vi "DisplayPanel.vi"() -> ()   [LabVIEW 2013]
uses:
  MvLVLib/MvCameraControl.lvlib
panel:
  in  "TimerTriggerActivation":u16(ring) items=["RisingEdge", "FallingEdge", "AnyEdge", "LevelHigh", "LevelLow"]
  in  "TimerTriggerSoftware":bool
  in  "TimerTriggerSource":u16(ring) items=["Off", "OptoCoupledInput0", "OptoCoupledInput1", "OptoCoupledInput2", "OptoCoupledInput3", "RS422diffInput0", "RS422diffInput1", "RS422diffInput2", "RS422diffInput3", "TTLInput0", "TTLInput1", "TTLInput2", "TTLInput3", "Timer0Active", "Timer1Active", "Timer2Active", "Timer3Active", "Encoder0", "Encoder1", "SoftwareSignal0", "Continuous"]
  in  "TimerFrequency":u32
  in  "TimerDelay":u32
  in  "TimerDuration":u32
  in  "TimerSelector":u16(ring) items=["Timer0", "Timer1", "Timer2", "Timer3"]
  in  "Interface List":u16(ring)
  out "handle":u64 format="%x"
  in  "Close Interface":bool
  in  "Open Interface":bool
  in  "Enum Interface":bool
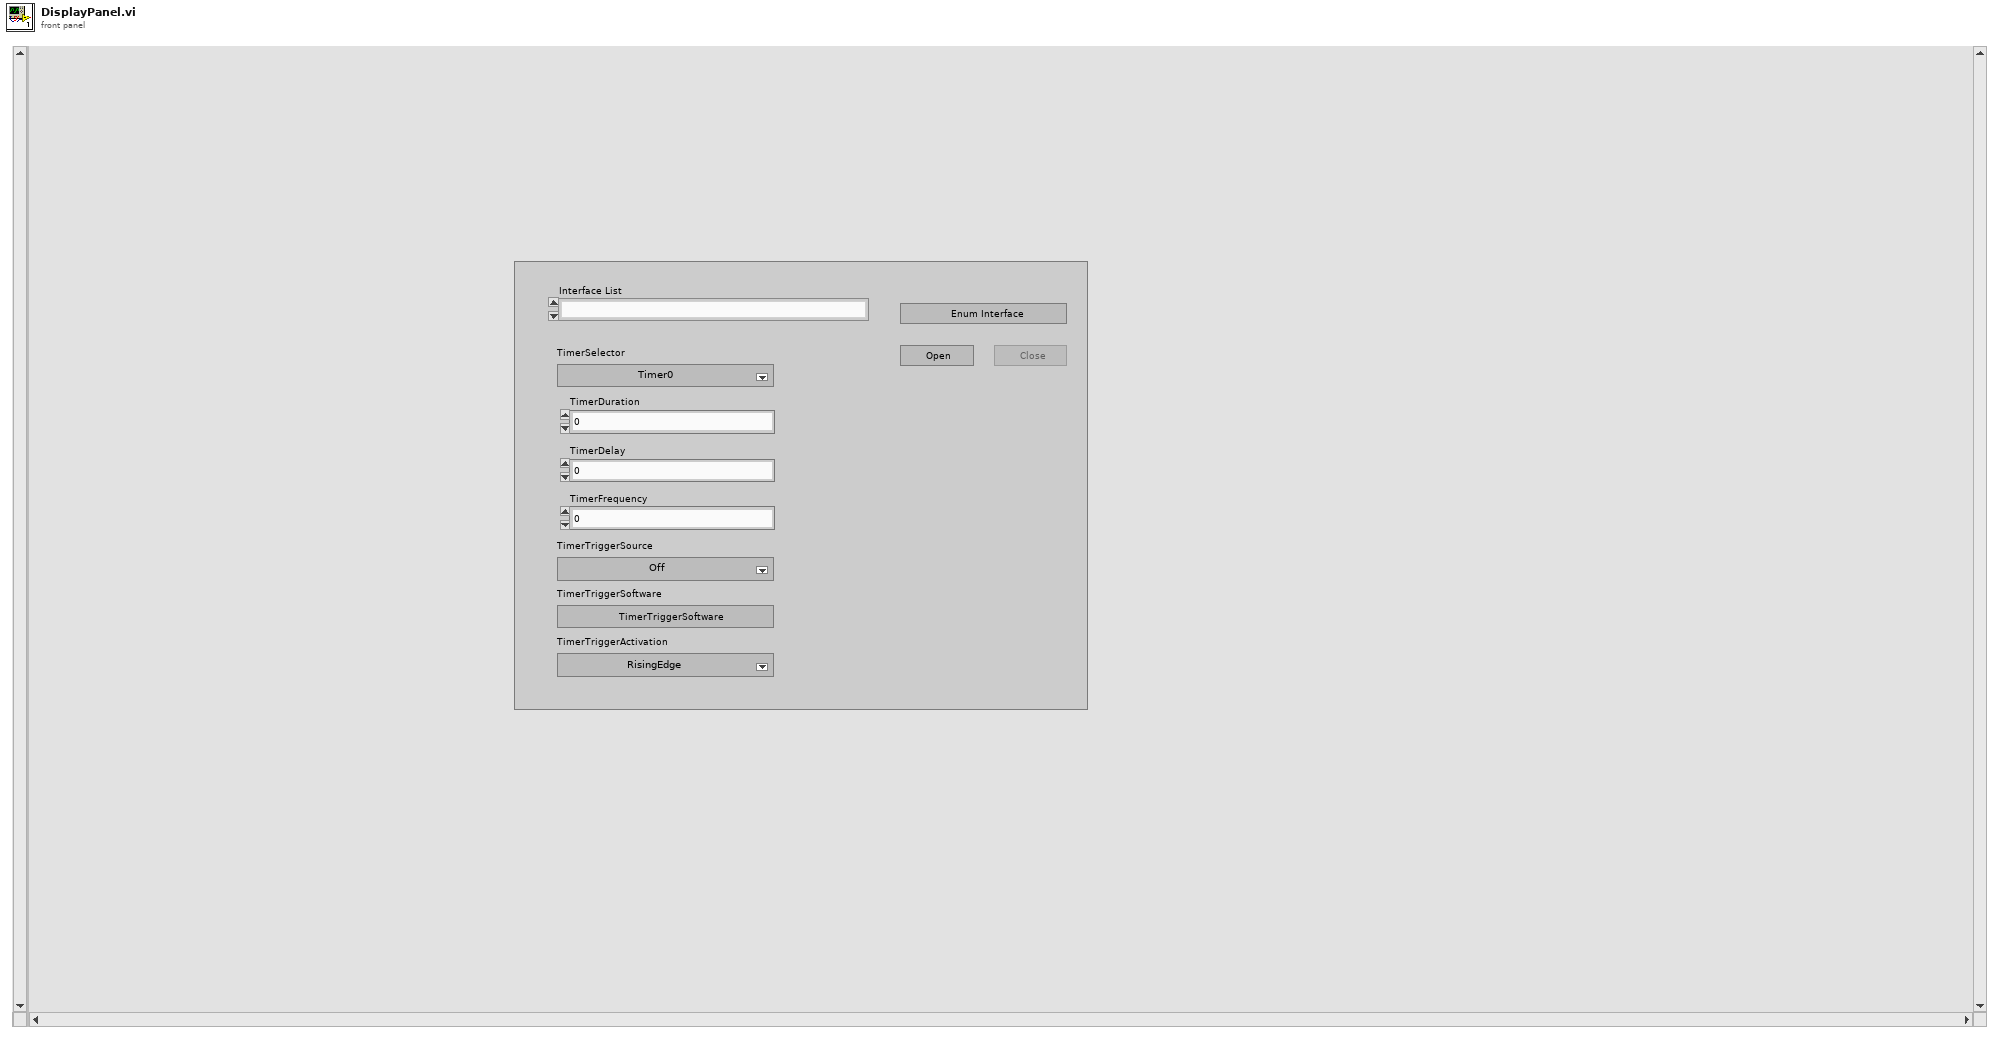
[diagram p1: front panel]
types:
  T1 = enum8{"Enabled", "Disabled", "Disabled and Grayed Out"}
  T2 = cluster{"nTLayerType":u32, "nPCIEInfo":u32, "chInterfaceID":string, "chDisplayName":string, "chSerialNumber":string, "chModelName":string, "chManufacturer":string, "chDeviceVersion":string, "chUserDefinedName":string}[]
  T3 = cluster{"nCurValue":u32, "nSupportedNum":u32, "nSupportValue":u32[], "nReserved[0]":u32, "nReserved[1]":u32, "nReserved[2]":u32, "nReserved[3]":u32}
  T4 = cluster{"nValue":u32, "chSymbolic":string, "nReserved[0]":u32, "nReserved[1]":u32, "nReserved[2]":u32, "nReserved[3]":u32}
  T5 = cluster{"nCurValue":u32, "nMax":u32, "nMin":u32, "nInc":u32, "nReserved[0]":u32, "nReserved[1]":u32, "nReserved[2]":u32, "nReserved[3]":u32}
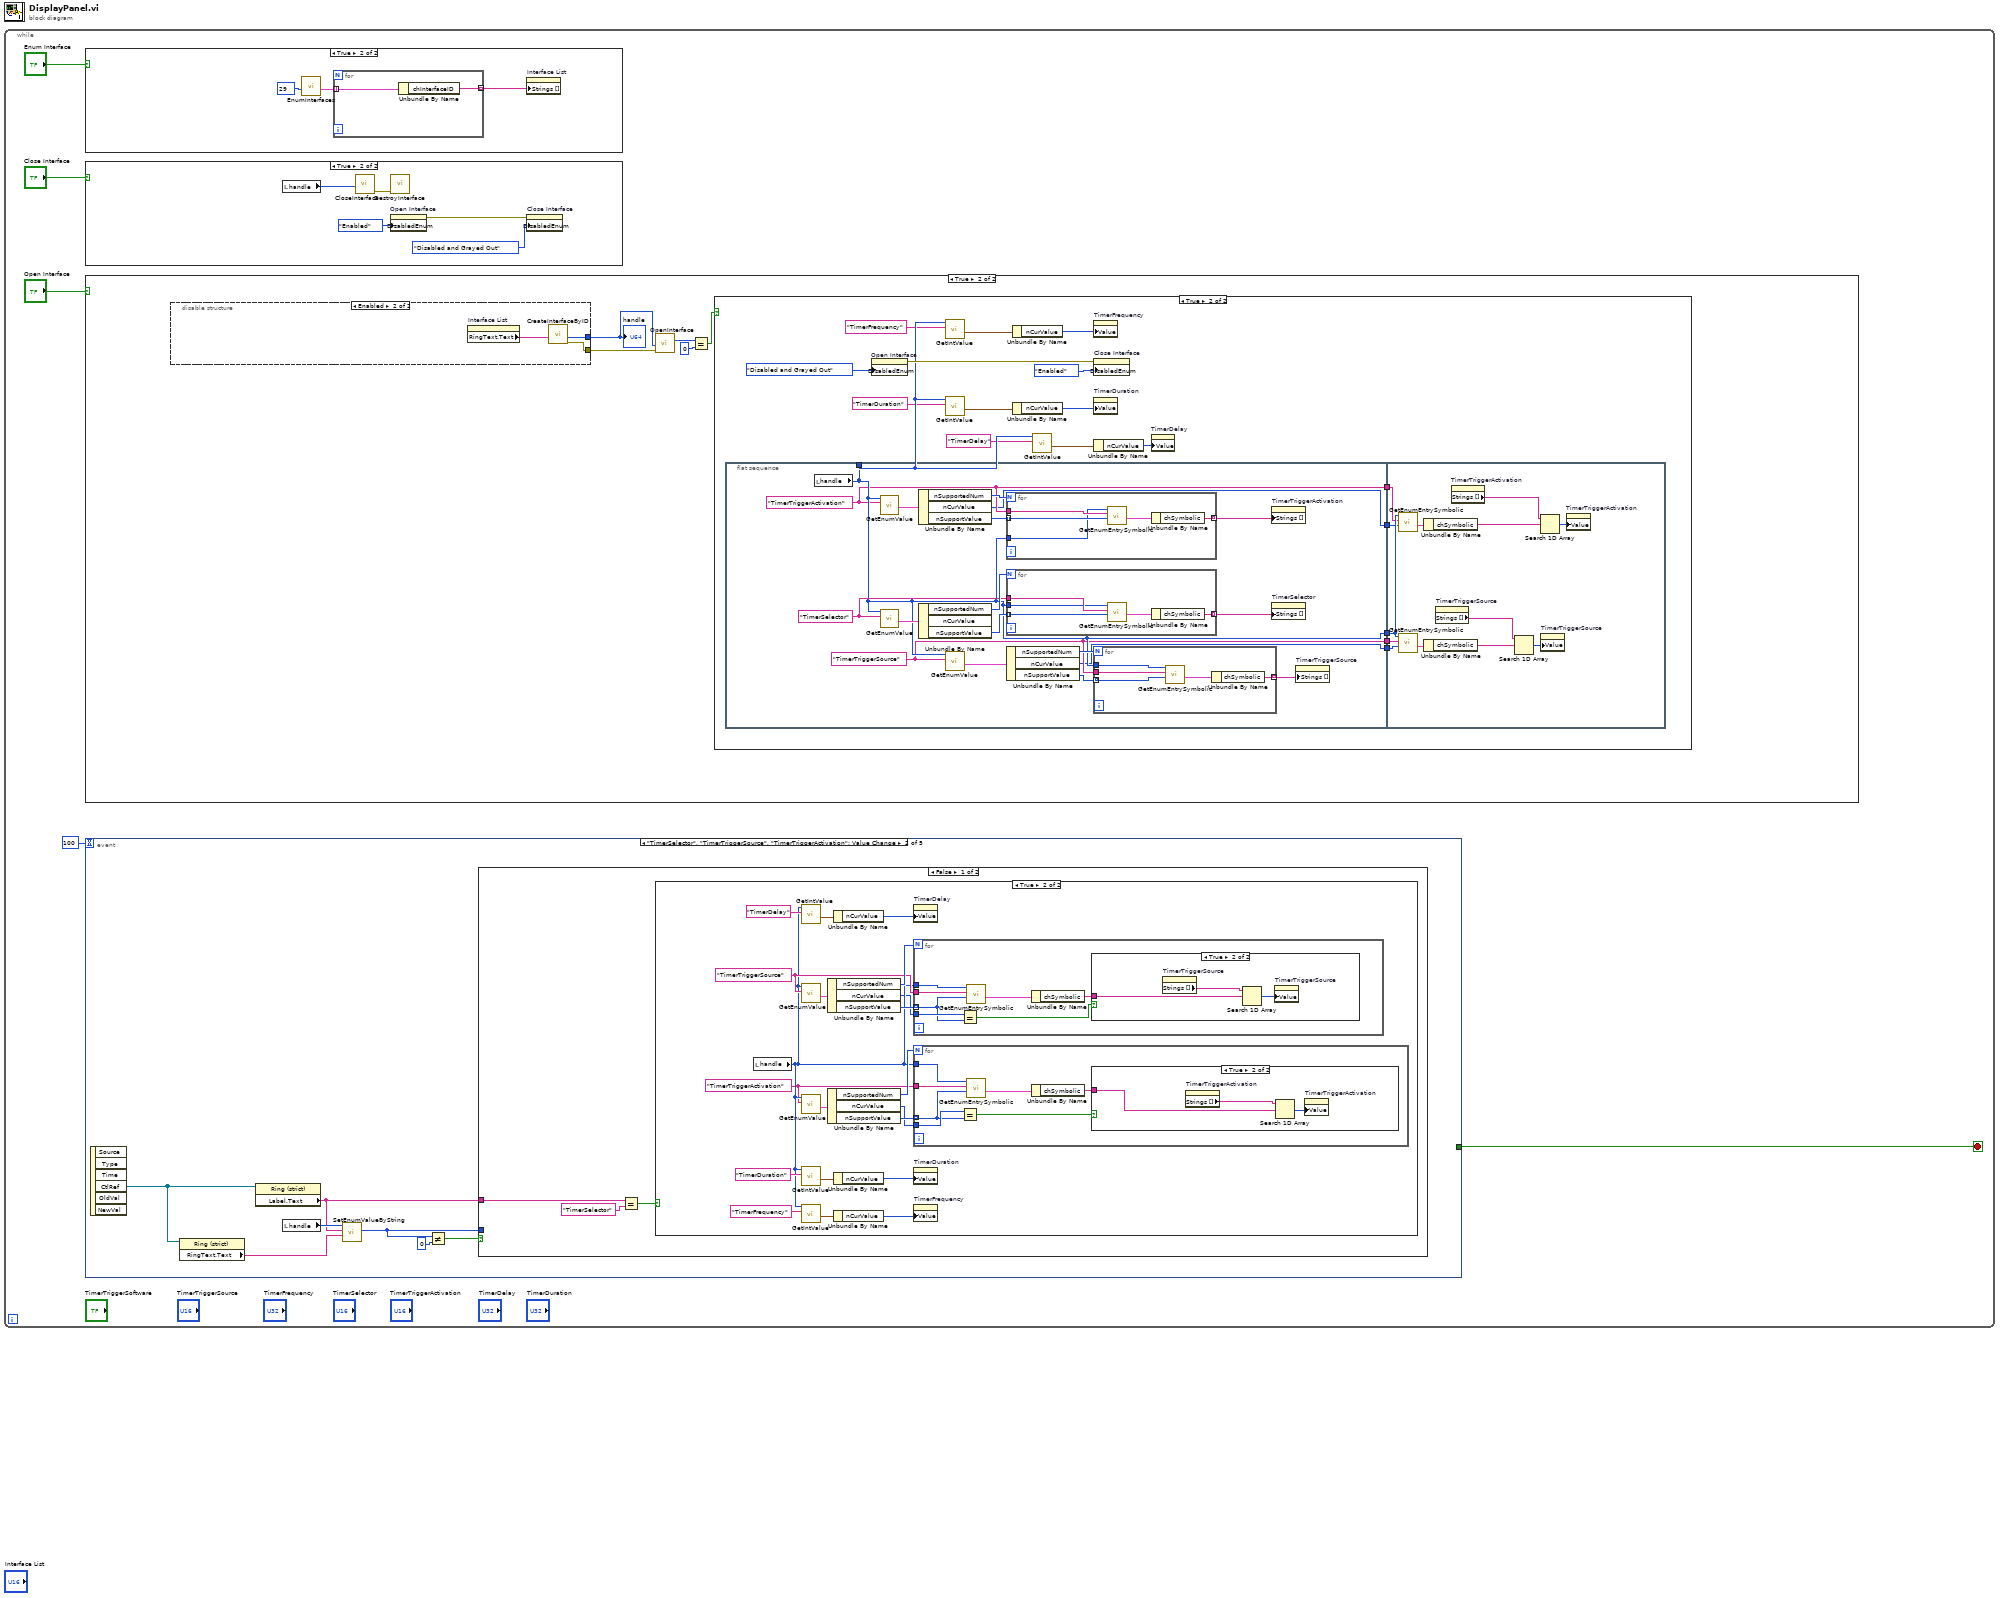
[diagram p0: block diagram]
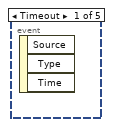
[diagram p2: hidden frame]
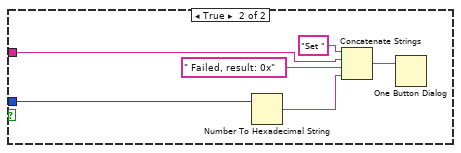
[diagram p6: hidden frame]
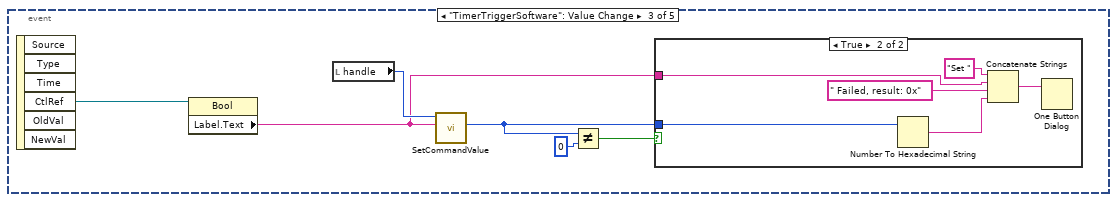
[diagram p7: hidden frame]
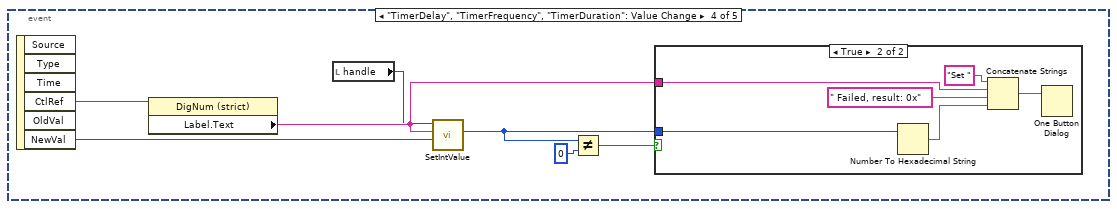
[diagram p9: hidden frame]
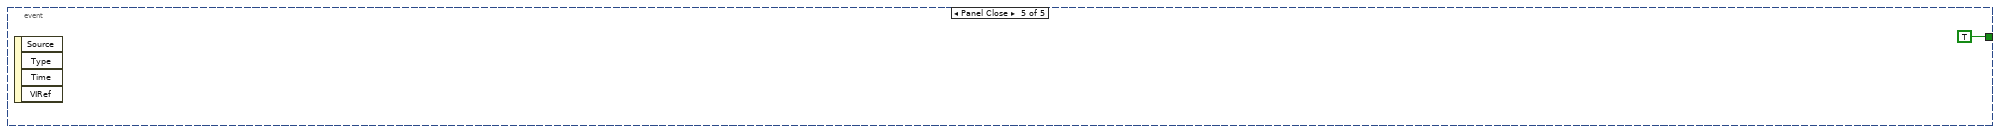
[diagram p11: hidden frame]
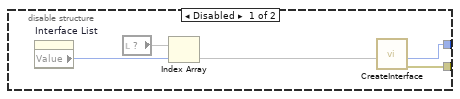
[diagram p14: hidden frame]
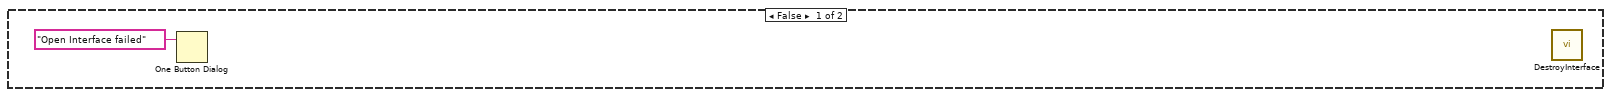
[diagram p15: hidden frame]
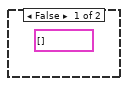
[diagram p16: hidden frame]
diagram:
  n1 = while {
    stop <- w2 stop-if-true
    n2 = case shown="True" "Enum Interface" {
      frame False {
        (unwired) T2 [] ("pInterfaceInfoList")
      }
      frame True {
        n3 = call "EnumInterfaces.vi"("nTLayerType"=u32 29) -> ("pInterfaceInfoList"=w171:T2)  [unwired: 8 in, 2 out]
        n4 = for {
          tunnel: w171 -> [w175] mode=indexing
          tunnel: [w174] -> w172 mode=indexing
          n5 = Unbundle By Name(w175) -> ("chInterfaceID"=w174:string)
        }
        n6 = property on="Interface List" class="Ring (strict)"("Strings []"=w172) -> ()  [unwired: 2 in, 2 out]
      }
    }
    n7 = case shown="True" "Close Interface" {
      frame False {
      }
      frame True {
        n8 = local read "handle"() -> (w89:u64)
        n9 = call "CloseInterface.vi"("handle"=w89) -> ("error out"=w92:errorcluster)  [unwired: 9 in, 1 out]
        n10 = call "DestroyInterface.vi"("error in (no error)"=w92) -> ()  [unwired: 9 in, 2 out]
        n11 = property on="Open Interface" class="Bool"("DisabledEnum"=T1."Enabled" ("Disabled")) -> (error out=w91:errorcluster)  [unwired: 2 in, 1 out]
        n12 = property on="Close Interface" class="Bool"(error in=w91, "DisabledEnum"=T1."Disabled and Grayed Out" ("Disabled")) -> ()  [unwired: 1 in, 2 out]
      }
    }
    n13 = case shown="True" "Open Interface" {
      frame False {
      }
      frame True {
        n14 = disable-structure shown="Enabled" {
          disable-tunnel: [w101 w105] -> w97
          disable-tunnel: [w100 w104] -> w93
          frame Disabled {
            n15 = property on="Interface List" class="Ring (strict)"() -> ("Value"=w102:u16)  [unwired: 2 in, 2 out]
            n16 = local read item#-1() -> (w99)
            n17 = Index Array(array=w99, index=w102) -> (element=w98)
            n18 = call "CreateInterface.vi"("InterfaceInfo"=w98) -> ("error out"=w101:errorcluster, "handle"=w100:i64)  [unwired: 8 in, 1 out]
          }
          frame Enabled {
            n19 = property on="Interface List" class="Ring (strict)"() -> ("RingText.Text"=w103:string)  [unwired: 2 in, 2 out]
            n20 = call "CreateInterfaceByID.vi"("pInterfaceID"=w103) -> ("error out"=w105:errorcluster, "handle"=w104:i64)  [unwired: 8 in, 1 out]
          }
        }
        "handle" <- w93
        n21 = call "OpenInterface.vi"("error in (no error)"=w97, "handle"=w93) -> ("return type"=w94:i32)  [unwired: 8 in, 1 out]
        n22 = Equal?(x=w94, y=u64 0) -> (x = y?=w95:bool)
        n23 = case shown="True" w95 {
          frame False {
            n24 = One Button Dialog(message="Open Interface failed") -> ()  [unwired: 1 in, 1 out]
            n25 = call "DestroyInterface.vi"() -> ()  [unwired: 10 in, 2 out]
          }
          frame True {
            n26 = flat-sequence {
              tunnel: [w129] -> w121
              tunnel: [w129] -> w111
              tunnel: [w128] -> w110
              tunnel: [w127] -> w109
              tunnel: [w126] -> w108
              tunnel: [w125] -> w107
              tunnel: w111 -> [w160]
              tunnel: w110 -> [w170]
              tunnel: w109 -> [w169]
              tunnel: w108 -> [w159]
              tunnel: w107 -> [w158]
              frame #0 {
                w126 = "TimerTriggerActivation" ("strKey")
                w128 = "TimerTriggerSource" ("strKey")
                w139 = "TimerSelector" ("strKey")
                n27 = local read "handle"() -> (w129:u64)
                n28 = call "GetEnumValue.vi"("strKey"=w126, "handle"=w129) -> ("pEnumValue out"=w132:T3)  [unwired: 6 in, 3 out]
                n29 = call "GetEnumValue.vi"("strKey"=w139, "handle"=w129) -> ("pEnumValue out"=w140:T3)  [unwired: 6 in, 3 out]
                n30 = Unbundle By Name(w132) -> ("nSupportedNum"=w130:u32, "nCurValue"=w125:u32, "nSupportValue"=w133:u32[])
                n31 = Unbundle By Name(w140) -> ("nSupportedNum"=w141:u32, "nSupportValue"=w138:u32[])  [unwired: 1 out]
                n32 = call "GetEnumValue.vi"("strKey"=w128, "handle"=w129) -> ("pEnumValue out"=w136:T3)  [unwired: 6 in, 3 out]
                n33 = for {
                  N: w130 -> [_]
                  tunnel: w126 -> [w147]
                  tunnel: [w145] -> w131 mode=indexing
                  tunnel: w133 -> [w144] mode=indexing
                  tunnel: w129 -> [w143]
                  n34 = call "GetEnumEntrySymbolic.vi"("nValue"=w144, "strKey"=w147, "handle"=w143) -> ("EnumEntry"=w146:T4)  [unwired: 5 in, 3 out]
                  n35 = Unbundle By Name(w146) -> ("chSymbolic"=w145:string)
                }
                n36 = for {
                  N: w141 -> [_]
                  tunnel: w139 -> [w157]
                  tunnel: w129 -> [w156]
                  tunnel: [w154] -> w142 mode=indexing
                  tunnel: w138 -> [w153] mode=indexing
                  n37 = call "GetEnumEntrySymbolic.vi"("nValue"=w153, "strKey"=w157, "handle"=w156) -> ("EnumEntry"=w155:T4)  [unwired: 5 in, 3 out]
                  n38 = Unbundle By Name(w155) -> ("chSymbolic"=w154:string)
                }
                n39 = Unbundle By Name(w136) -> ("nSupportedNum"=w134:u32, "nCurValue"=w127:u32, "nSupportValue"=w137:u32[])
                n40 = for {
                  N: w134 -> [_]
                  tunnel: w128 -> [w152]
                  tunnel: [w150] -> w135 mode=indexing
                  tunnel: w137 -> [w149] mode=indexing
                  tunnel: w129 -> [w148]
                  n41 = call "GetEnumEntrySymbolic.vi"("nValue"=w149, "strKey"=w152, "handle"=w148) -> ("EnumEntry"=w151:T4)  [unwired: 5 in, 3 out]
                  n42 = Unbundle By Name(w151) -> ("chSymbolic"=w150:string)
                }
                n43 = property on="TimerTriggerActivation" class="Ring (strict)"("Strings []"=w131) -> ()  [unwired: 2 in, 2 out]
                n44 = property on="TimerSelector" class="Ring (strict)"("Strings []"=w142) -> ()  [unwired: 2 in, 2 out]
                n45 = property on="TimerTriggerSource" class="Ring (strict)"("Strings []"=w135) -> ()  [unwired: 2 in, 2 out]
              }
              frame #1 {
                n46 = call "GetEnumEntrySymbolic.vi"("nValue"=w158, "strKey"=w159, "handle"=w160) -> ("EnumEntry"=w163:T4)  [unwired: 5 in, 3 out]
                n47 = call "GetEnumEntrySymbolic.vi"("nValue"=w169, "strKey"=w170, "handle"=w160) -> ("EnumEntry"=w166:T4)  [unwired: 5 in, 3 out]
                n48 = Unbundle By Name(w163) -> ("chSymbolic"=w164:string)
                n49 = Unbundle By Name(w166) -> ("chSymbolic"=w165:string)
                n50 = property on="TimerTriggerSource" class="Ring (strict)"() -> ("Strings []"=w167:string[])  [unwired: 2 in, 2 out]
                n51 = property on="TimerTriggerActivation" class="Ring (strict)"() -> ("Strings []"=w162:string[])  [unwired: 2 in, 2 out]
                n52 = Search 1D Array(1D array=w167, element=w165) -> (index of element=w168:i32)  [unwired: 1 in]
                n53 = Search 1D Array(1D array=w162, element=w164) -> (index of element=w161:i32)  [unwired: 1 in]
                n54 = property on="TimerTriggerSource" class="Ring (strict)"("Value"=w168) -> ()  [unwired: 2 in, 2 out]
                n55 = property on="TimerTriggerActivation" class="Ring (strict)"("Value"=w161) -> ()  [unwired: 2 in, 2 out]
              }
            }
            n56 = property on="Open Interface" class="Bool"("DisabledEnum"=T1."Disabled and Grayed Out" ("Disabled")) -> (error out=w123:errorcluster)  [unwired: 2 in, 1 out]
            n57 = call "GetIntValue.vi"("strKey"="TimerFrequency", "handle"=w121) -> ("pIntValue out"=w113:T5)  [unwired: 6 in, 3 out]
            n58 = call "GetIntValue.vi"("strKey"="TimerDuration", "handle"=w121) -> ("pIntValue out"=w119:T5)  [unwired: 6 in, 3 out]
            n59 = Unbundle By Name(w113) -> ("nCurValue"=w112:u32)
            n60 = Unbundle By Name(w119) -> ("nCurValue"=w118:u32)
            n61 = call "GetIntValue.vi"("strKey"="TimerDelay", "handle"=w121) -> ("pIntValue out"=w116:T5)  [unwired: 6 in, 3 out]
            n62 = property on="TimerFrequency" class="DigNum (strict)"("Value"=w112) -> ()  [unwired: 2 in, 2 out]
            n63 = property on="Close Interface" class="Bool"(error in=w123, "DisabledEnum"=T1."Enabled" ("Disabled")) -> ()  [unwired: 1 in, 2 out]
            n64 = property on="TimerDuration" class="DigNum (strict)"("Value"=w118) -> ()  [unwired: 2 in, 2 out]
            n65 = Unbundle By Name(w116) -> ("nCurValue"=w117:u32)
            n66 = property on="TimerDelay" class="DigNum (strict)"("Value"=w117) -> ()  [unwired: 2 in, 2 out]
          }
        }
      }
    }
    n67 = event shown="[1] \"TimerSelector\", \"TimerTriggerSource\", \"TimerTriggerActivation\": Value Change" {
      selector: _ -> [_ _ _ _ _]
      dyn-events: _ -> [_ _ _ _ _]
      timeout: 100 -> [_ _ _ _ _]
      tunnel: [_ _ _ _ TRUE] -> w2
      event Timeout {
        n68 = event-data() -> ()  [unwired: 1 in, 3 out]
      }
      event "TimerSelector", "TimerTriggerSource", "TimerTriggerActivation": Value Change {
        n69 = event-data() -> ("CtlRef"=w10:refnum<vi>)  [unwired: 1 in, 5 out]
        n70 = property class="Ring (strict)"(reference=w10) -> ("RingText.Text"=w11:string)  [unwired: 1 in, 2 out]
        n71 = property class="Ring (strict)"(reference=w10) -> ("Label.Text"=w7:string)  [unwired: 1 in, 2 out]
        n72 = local read "handle"() -> (w12:u64)
        n73 = call "SetEnumValueByString.vi"("strValue"=w11, "strKey"=w7, "handle"=w12) -> ("function return"=w6:i32)  [unwired: 6 in, 2 out]
        n74 = Not Equal?(x=w6, y=0) -> (x != y?=w8:bool)
        n75 = case shown="False" w8 {
          tunnel: w7 -> [w15 w60]
          tunnel: w6 -> [_ w59]
          frame False {
            n76 = Equal?(x=w15, y="TimerSelector") -> (x = y?=w13:bool)
            n77 = case shown="True" w13 {
              frame False {
              }
              frame True {
                w18 = "TimerTriggerActivation" ("strKey")
                w21 = "TimerTriggerSource" ("strKey")
                n78 = local read "handle"() -> (w19:u64)
                n79 = call "GetIntValue.vi"("strKey"="TimerDelay", "handle"=w19) -> ("pIntValue out"=w28:T5)  [unwired: 6 in, 3 out]
                n80 = call "GetEnumValue.vi"("strKey"=w21, "handle"=w19) -> ("pEnumValue out"=w22:T3)  [unwired: 6 in, 3 out]
                n81 = call "GetEnumValue.vi"("strKey"=w18, "handle"=w19) -> ("pEnumValue out"=w34:T3)  [unwired: 6 in, 3 out]
                n82 = call "GetIntValue.vi"("strKey"="TimerDuration", "handle"=w19) -> ("pIntValue out"=w25:T5)  [unwired: 6 in, 3 out]
                n83 = call "GetIntValue.vi"("strKey"="TimerFrequency", "handle"=w19) -> ("pIntValue out"=w31:T5)  [unwired: 6 in, 3 out]
                n84 = Unbundle By Name(w22) -> ("nSupportedNum"=w23:u32, "nCurValue"=w16:u32, "nSupportValue"=w20:u32[])
                n85 = Unbundle By Name(w34) -> ("nSupportedNum"=w35:u32, "nCurValue"=w17:u32, "nSupportValue"=w33:u32[])
                n86 = Unbundle By Name(w28) -> ("nCurValue"=w27:u32)
                n87 = Unbundle By Name(w25) -> ("nCurValue"=w26:u32)
                n88 = Unbundle By Name(w31) -> ("nCurValue"=w32:u32)
                n89 = property on="TimerDelay" class="DigNum (strict)"("Value"=w27) -> ()  [unwired: 2 in, 2 out]
                n90 = for {
                  N: w23 -> [_]
                  tunnel: w21 -> [w52]
                  tunnel: w19 -> [w51]
                  tunnel: w20 -> [w47] mode=indexing
                  tunnel: w16 -> [w48]
                  n91 = Equal?(x=w48, y=w47) -> (x = y?=w49:bool)
                  n92 = call "GetEnumEntrySymbolic.vi"("nValue"=w47, "strKey"=w52, "handle"=w51) -> ("EnumEntry"=w50:T4)  [unwired: 5 in, 3 out]
                  n93 = Unbundle By Name(w50) -> ("chSymbolic"=w46:string)
                  n94 = case shown="True" w49 {
                    tunnel: w46 -> [_ w54]
                    frame False {
                    }
                    frame True {
                      n95 = property on="TimerTriggerSource" class="Ring (strict)"() -> ("Strings []"=w55:string[])  [unwired: 2 in, 2 out]
                      n96 = Search 1D Array(1D array=w55, element=w54) -> (index of element=w53:i32)  [unwired: 1 in]
                      n97 = property on="TimerTriggerSource" class="Ring (strict)"("Value"=w53) -> ()  [unwired: 2 in, 2 out]
                    }
                  }
                }
                n98 = for {
                  N: w35 -> [_]
                  tunnel: w18 -> [w42]
                  tunnel: w19 -> [w41]
                  tunnel: w33 -> [w37] mode=indexing
                  tunnel: w17 -> [w38]
                  n99 = Equal?(x=w38, y=w37) -> (x = y?=w39:bool)
                  n100 = call "GetEnumEntrySymbolic.vi"("nValue"=w37, "strKey"=w42, "handle"=w41) -> ("EnumEntry"=w40:T4)  [unwired: 5 in, 3 out]
                  n101 = Unbundle By Name(w40) -> ("chSymbolic"=w36:string)
                  n102 = case shown="True" w39 {
                    tunnel: w36 -> [_ w43]
                    frame False {
                    }
                    frame True {
                      n103 = property on="TimerTriggerActivation" class="Ring (strict)"() -> ("Strings []"=w44:string[])  [unwired: 2 in, 2 out]
                      n104 = Search 1D Array(1D array=w44, element=w43) -> (index of element=w45:i32)  [unwired: 1 in]
                      n105 = property on="TimerTriggerActivation" class="Ring (strict)"("Value"=w45) -> ()  [unwired: 2 in, 2 out]
                    }
                  }
                }
                n106 = property on="TimerDuration" class="DigNum (strict)"("Value"=w26) -> ()  [unwired: 2 in, 2 out]
                n107 = property on="TimerFrequency" class="DigNum (strict)"("Value"=w32) -> ()  [unwired: 2 in, 2 out]
              }
            }
          }
          frame True {
            n108 = Number To Hexadecimal String(2:w59) -> (0:w57:string)  [unwired: 1 in]
            n109 = Concatenate Strings("Set " ("message"), w60, " Failed, result: 0x" ("string"), w57) -> (w56:string)
            n110 = One Button Dialog(message=w56) -> ()  [unwired: 1 in, 1 out]
          }
        }
      }
      event "TimerTriggerSoftware": Value Change {
        n111 = event-data() -> ("CtlRef"=w66:refnum<vi>)  [unwired: 1 in, 5 out]
        n112 = property class="Bool"(reference=w66) -> ("Label.Text"=w62:string)  [unwired: 1 in, 2 out]
        n113 = local read "handle"() -> (w65:u64)
        n114 = call "SetCommandValue.vi"("strValue"=w62, "handle"=w65) -> ("function return"=w63:i32)  [unwired: 7 in, 2 out]
        n115 = Not Equal?(x=w63, y=0) -> (x != y?=w67:bool)
        n116 = case shown="True" w67 {
          tunnel: w63 -> [_ w69]
          tunnel: w62 -> [_ w68]
          frame False {
          }
          frame True {
            n117 = Number To Hexadecimal String(2:w69) -> (0:w71:string)  [unwired: 1 in]
            n118 = Concatenate Strings("Set " ("message"), w68, " Failed, result: 0x" ("string"), w71) -> (w70:string)
            n119 = One Button Dialog(message=w70) -> ()  [unwired: 1 in, 1 out]
          }
        }
      }
      event "TimerDelay", "TimerFrequency", "TimerDuration": Value Change {
        n120 = event-data() -> ("CtlRef"=w75:refnum<vi>, "NewVal"=w74:u32)  [unwired: 1 in, 4 out]
        n121 = property class="DigNum (strict)"(reference=w75) -> ("Label.Text"=w80:string)  [unwired: 1 in, 2 out]
        n122 = local read "handle"() -> (w78:u64)
        n123 = call "SetIntValue.vi"("nValue"=w74, "strKey"=w80, "handle"=w78) -> ("function return"=w79:i32)  [unwired: 6 in, 2 out]
        n124 = Not Equal?(x=w79, y=0) -> (x != y?=w77:bool)
        n125 = case shown="True" w77 {
          tunnel: w79 -> [_ w82]
          tunnel: w80 -> [_ w81]
          frame False {
          }
          frame True {
            n126 = Number To Hexadecimal String(2:w82) -> (0:w84:string)  [unwired: 1 in]
            n127 = Concatenate Strings("Set " ("message"), w81, " Failed, result: 0x" ("string"), w84) -> (w83:string)
            n128 = One Button Dialog(message=w83) -> ()  [unwired: 1 in, 1 out]
          }
        }
      }
      event Panel Close {
        n129 = event-data() -> ()  [unwired: 1 in, 4 out]
      }
    }
  }
